vi "Channel Probe.vi"(2 "channelOp":T1, 3 "EventMessengerMData":refnum<class "EventMessengerMData.lvclass">) -> (1 "EventMessengerMData out":refnum<class "EventMessengerMData.lvclass">)   [LabVIEW 2019, in "Event MessengerM.lvlib"]
doc: "Displays the status of the channel as the channel is modified by the various endpoints and gives the user ways to pause the application using the channel."
uses:
  Event MessengerM.lvlib
  EventMessengerMData.lvclass
  ChannelOp.ctl
panel:
  in  "subchannel":i32
  in  "Details":string="Details"
  in  "Write Count":string="Write Count"
  out "Details":string
  in  "Pause when aborted":bool
  in  "Pause when last element written":bool
  out "Details":string
  in  "Play":bool
  out "Aborted?":bool
  out "Last element written?":bool
  in  "Pause":bool
  # "Details"
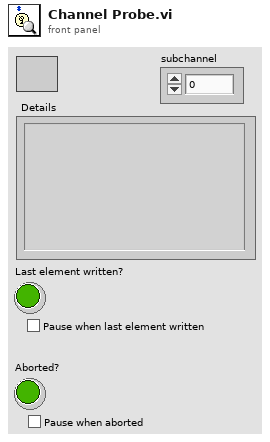
[diagram p1: front panel]
types:
  T1 = typedef "Event MessengerM.lvlib/ChannelOp.ctl" = enum16{"init", "write", "register", "replicate", "probe"}
  T2 = enum32{"Invalid", "Standard", "Closed", "Hidden", "Minimized", "Maximized"}
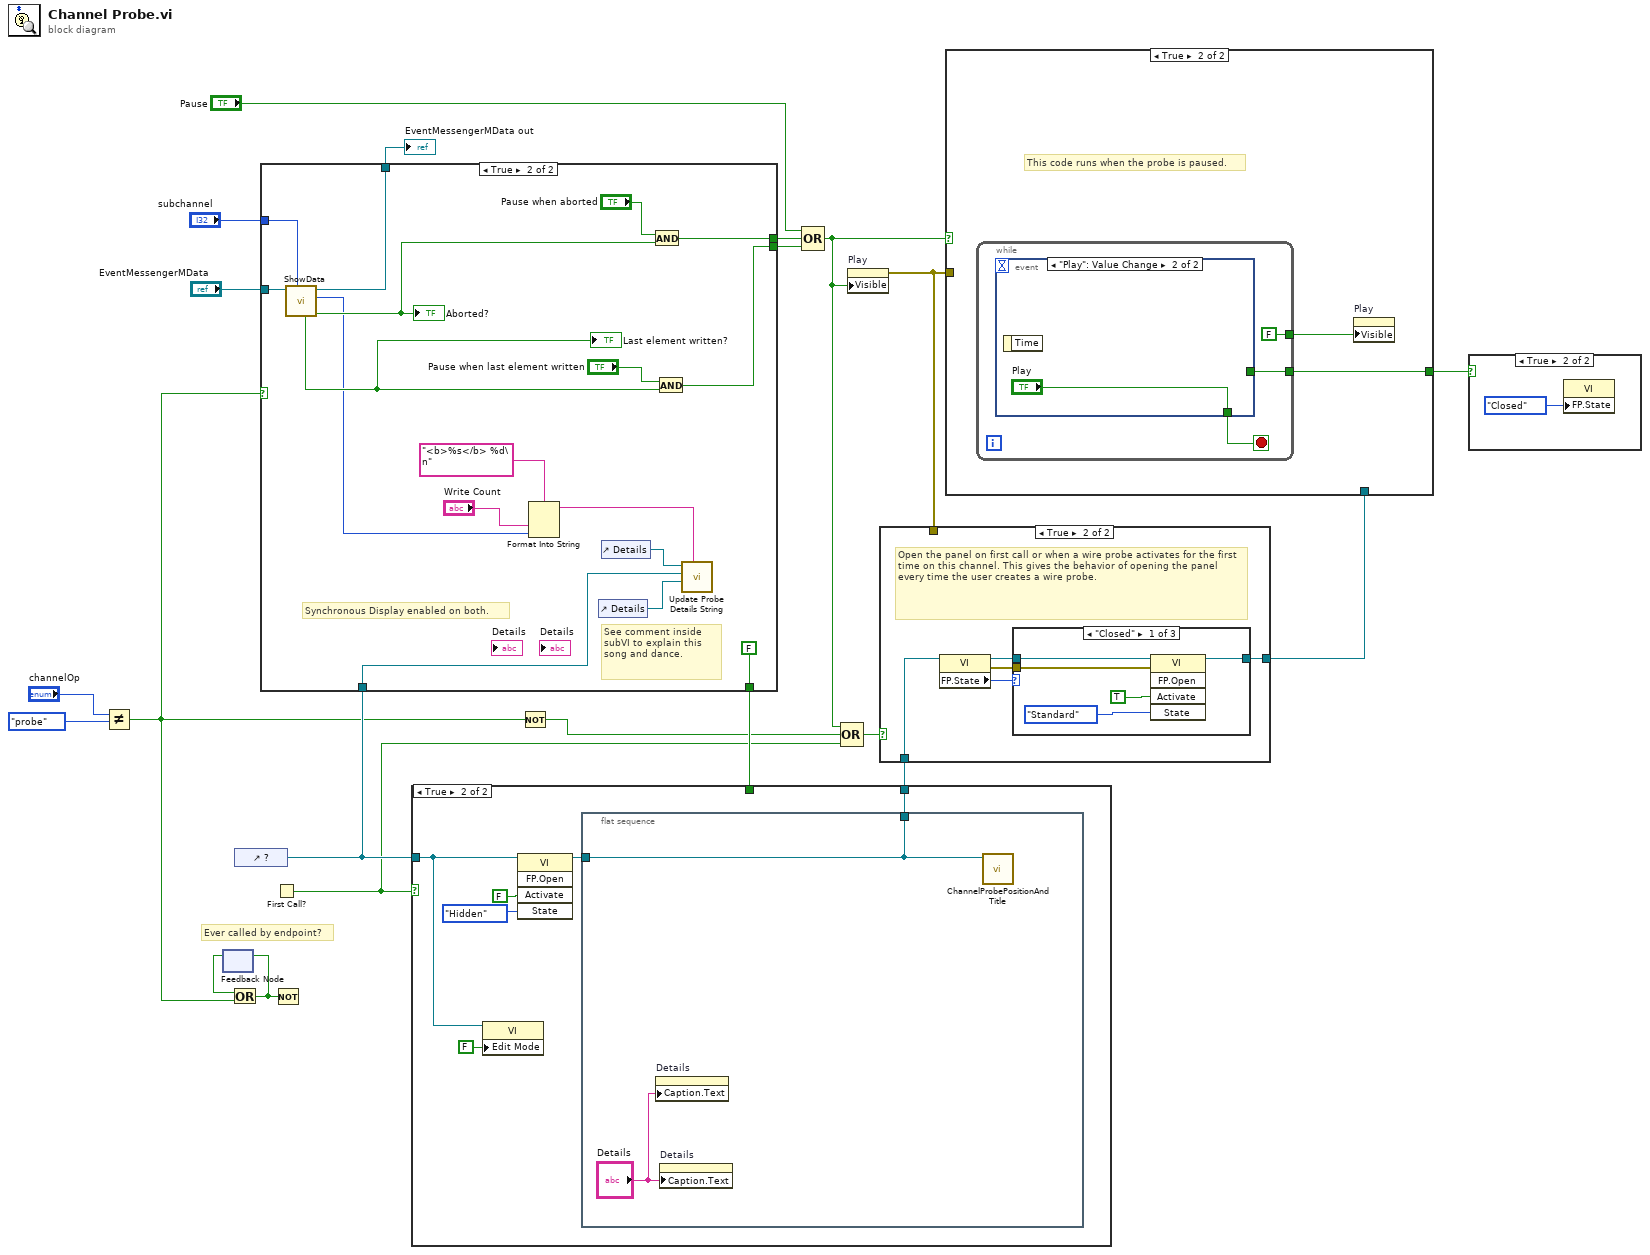
[diagram p0: block diagram]
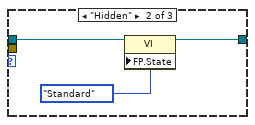
[diagram p3: hidden frame]
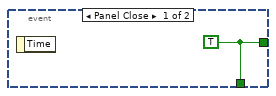
[diagram p8: hidden frame]
diagram:
  # "Ever called by endpoint?"
  n1 = Not Equal?(x="channelOp", y=ChannelOp."probe" ("channelOp")) -> (x != y?=w5:bool)
  n2 = feedback #1() -> (w15:bool)  [unwired: 1 in]
  n3 = Or(x=w15, y=w5) -> (x .or. y?=w14:bool)
  n4 = feedback-in #1(w14) -> ()
  n5 = control-ref of="?"() -> (w16:refnum<vi>)
  n6 = case shown="True" w5 {
    tunnel: "EventMessengerMData" -> [w22 w39]
    tunnel: [_ w36] -> w20
    tunnel: [_ w35] -> w18
    tunnel: [_ FALSE ("always false")] -> w17
    tunnel: w16 -> [_ w33]
    tunnel: [w22 w28] -> w3
    tunnel: "subchannel" -> [_ w23]
    frame False {
    }
    frame True {
      # "See comment inside subVI to explain this song and dance."
      # "Synchronous Display enabled on both."
      n7 = call "ShowData.vi"("subchannel"=w23, "data in"=w39) -> ("aborted?"=w26:bool, "write count"=w25:u32, "data out"=w28:refnum<class "EventMessengerMData.lvclass">, "last element?"=w27:bool)  [unwired: 6 in]
      "Last element written?" <- w27
      "Aborted?" <- w26
      n8 = Format Into String(format string="<b>%s</b> %d\n", "Write Count", w25) -> (resulting string=w24:string)  [unwired: 2 in, 1 out]
      n9 = control-ref of="Details"() -> (w34:refnum<vi>)
      n10 = control-ref of="Details"() -> (w32:refnum<vi>)
      n11 = And(x="Pause when aborted", y=w26) -> (x .and. y?=w36:bool)
      n12 = And(x="Pause when last element written", y=w27) -> (x .and. y?=w35:bool)
      n13 = call <resource>:"Update Probe Details String.vi"("String"=w24, "Details 1"=w34, "VI Reference"=w33, "Details 2"=w32) -> ()  [unwired: 8 in]
    }
  }
  "EventMessengerMData out" <- w3
  n14 = First Call?() -> (First Call?: T/F=w8:bool)
  n15 = Not(x=w14) -> ()  [unwired: 1 out]
  n16 = case shown="True" w8 {
    tunnel: [w40 w46] -> w12
    tunnel: w16 -> [w40 w42]
    tunnel: w17 -> [_ _]
    frame False {
    }
    frame True {
      n17 = property class="VI"(reference=w42, "Edit Mode"=FALSE ("Edit Mode On Open")) -> ()  [unwired: 1 in, 2 out]
      n18 = invoke class="VI" method="FP.Open"(reference=w42, "Activate"=FALSE ("Activate?"), "State"=T2."Hidden") -> (reference out=w43:refnum<vi>)  [unwired: 2 in, 4 out]
      n19 = flat-sequence {
        tunnel: [w47] -> w46
        tunnel: w43 -> [w47]
        frame #0 {
          n20 = property on="Details" class="Str"("Caption.Text"="Details") -> ()  [unwired: 2 in, 2 out]
          n21 = property on="Details" class="Str"("Caption.Text"="Details") -> ()  [unwired: 2 in, 2 out]
          n22 = call <resource>:"ChannelProbePositionAndTitle.vi"("VI in"=w47) -> ()  [unwired: 9 in, 2 out]
        }
      }
    }
  }
  n23 = Not(x=w5) -> (.not. x?=w9:bool)
  n24 = Compound Arithmetic op=OR("Pause", w20, w18) -> (w6:bool)
  n25 = Compound Arithmetic op=OR(w6, w9, w8) -> (w7:bool)
  n26 = property on="Play" class="Bool"("Visible"=w6) -> (error out=w11:errorcluster)  [unwired: 2 in, 1 out]
  n27 = case shown="True" w7 {
    tunnel: [w49 w51] -> w13
    tunnel: w12 -> [w49 w50]
    tunnel: w11 -> [_ _]
    frame False {
    }
    frame True {
      # "Open the panel on first call or when a wire probe activates for the first time on this channel. This gives the behavior of opening the panel every time the user creates a wire probe."
      n28 = property class="VI"(reference=w50) -> (reference out=w52:refnum<vi>, error out=w53:errorcluster, "FP.State"=w54:T2)  [unwired: 1 in]
      n29 = case shown="\"Closed\"" w54 {
        tunnel: w53 -> [w58 _ _]
        tunnel: w52 -> [w59 w62 w63]
        tunnel: [w55 w61 w63] -> w51
        frame "Closed" {
          n30 = invoke class="VI" method="FP.Open"(reference=w59, error in=w58, "Activate"=TRUE ("Activate?"), "State"=T2."Standard") -> (reference out=w55:refnum<vi>)  [unwired: 1 in, 4 out]
        }
        frame "Hidden" {
          n31 = property class="VI"(reference=w62, "FP.State"=T2."Standard" ("Front Panel Window:State")) -> (reference out=w61:refnum<vi>)  [unwired: 1 in, 1 out]
        }
        frame Default {
        }
      }
    }
  }
  n32 = case shown="True" w6 {
    tunnel: w13 -> [_ _]
    tunnel: [_ w65] -> w21
    tunnel: w11 -> [_ _]
    frame False {
    }
    frame True {
      # "This code runs when the probe is paused."
      n33 = while {
        tunnel: [w68] -> w65
        tunnel: [FALSE ("Visible")] -> w64
        stop <- w67 stop-if-true
        n34 = event shown="[1] \"Play\": Value Change" {
          selector: _ -> [_ _]
          dyn-events: _ -> [_ _]
          timeout: _ -> [_ _]
          tunnel: [w69 _] -> w68
          tunnel: [w69 "Play"] -> w67
          event Panel Close {
            w69 = TRUE
            n35 = event-data() -> ()  [unwired: 1 in, 1 out]
          }
          event "Play": Value Change {
            n36 = event-data() -> ()  [unwired: 1 in, 1 out]
          }
        }
      }
      n37 = property on="Play" class="Bool"("Visible"=w64) -> ()  [unwired: 2 in, 2 out]
    }
  }
  n38 = case shown="True" w21 {
    frame False {
    }
    frame True {
      n39 = property class="VI"("FP.State"=T2."Closed" ("Front Panel Window:State")) -> ()  [unwired: 2 in, 2 out]
    }
  }
